vi "Log Command.vi"(7 "Embedded Data Logger File Name":string, 8 "error in":errorcluster, 10 "Log Command":enum16{"Idle", "Open File", "Close File"}(ring), 11 "Embedded Data Logger System Tests in":refnum<class "Embedded Data Logger System Tests.lvclass">) -> (0 "error out":errorcluster, 3 "Embedded Data Logger System Tests out":refnum<class "Embedded Data Logger System Tests.lvclass">)   [LabVIEW 2018, in "Embedded Data Logger System Tests.lvclass"]
uses:
  Embedded Data Logger System Tests.lvclass
  C:/dev/niveristand-custom-device-testing-tools/VeriStandTestCase/VeriStandTestCase.lvclass
  <vilib>/NI Veristand/Execution/Workspace/NI VeriStand - Set Single Channel Value.vi
  <vilib>/NI Veristand/Execution/Workspace/NI_VS Workspace ExecutionAPI.lvlib
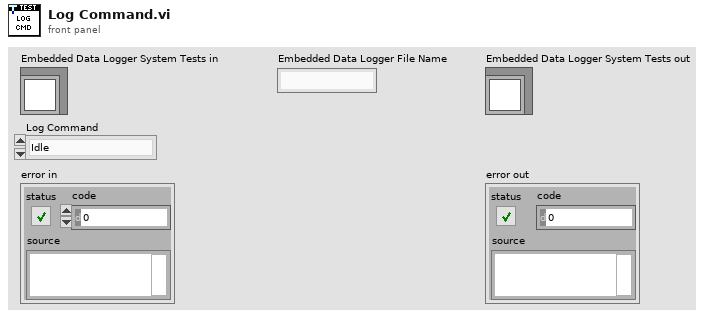
[diagram p1: front panel]
types:
  T1 = typedef "NI_VS Workspace ExecutionAPI.lvlib/WorkspaceAPI.ctl" = refnum<k24>
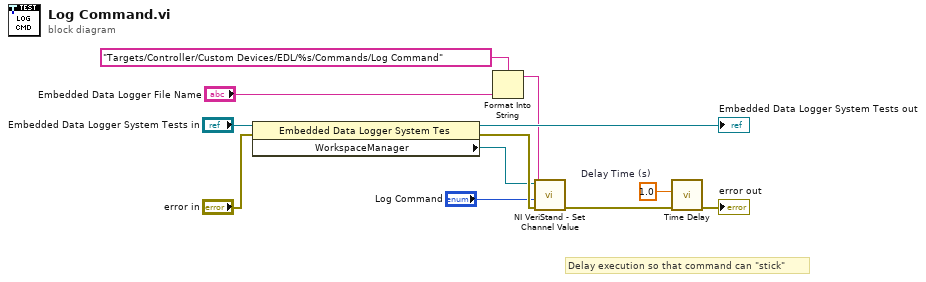
[diagram p0: block diagram]
diagram:
  w6 = 1.0  # Delay Time (s)
  # "Delay execution so that command can \"stick\""
  n1 = property class="Embedded Data Logger System Tes"(reference="Embedded Data Logger System Tests in", error in="error in") -> (reference out=→"Embedded Data Logger System Tests out":refnum<class "Embedded Data Logger System Tests.lvclass">, error out=w11:errorcluster, "WorkspaceManager"=w10:T1)
  n2 = Format Into String(format string="Targets/Controller/Custom Devices/EDL/%s/Commands/Log Command" ("Channel"), "Embedded Data Logger File Name") -> (resulting string=w3:string)  [unwired: 2 in, 1 out]
  n3 = call-poly <vilib>:"NI VeriStand - Set Channel Value.vi"("error in (no error)"=w11, "Value"="Log Command", "Channel"=w3, "WorkspaceManager in"=w10) -> ("error out"=w5:errorcluster)  [unwired: 6 in, 1 out]
  n4 = call "Time Delay"("error in (no error)"=w5, "Delay Time (s)"=w6) -> ("error out"=→"error out":errorcluster)  [unwired: 9 in]
